vi "ZPL Close.vi"(6 "error":errorcluster, 9 "VISA name":refnum<visa-resource-name>) -> (0 "error out":errorcluster)   [LabVIEW 2015]
doc: "This vi will add a checksum to any command string.\nThe format of the \"ChkSum Cmd\" output is:\n \"Command\" & \"Dollar Sign\" & \"Two Hex Digits\" & \"Carriage Return\"\n\nThe command is only formulated, it is not sent to the instrument."
panel:
  # "Lambda ZPLUS \n Serial Port\n  DC Power Supplies"
  # "Close Instrument Port"
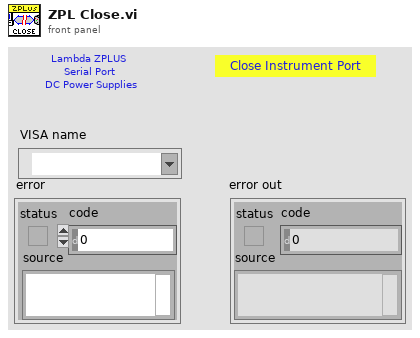
[diagram p1: front panel]
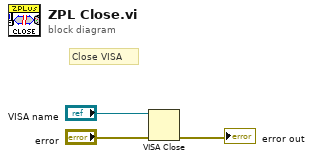
[diagram p0: block diagram]
diagram:
  # "Close VISA"
  n1 = VISA Close(VISA resource name="VISA name", error in (no error)="error") -> (error out=→"error out":errorcluster)
